vi "Calculate_Integrals.vi"(11 "SiPM Waveform":waveform(dbl)[](array[waveform])) -> (0 "Discrimination":string[](array[string]), 1 "Tail Integral":dbl[](array[numeric]), 2 "dt":dbl, 3 "Data Points":dbl[][](array[numeric]), 4 "Total Integral":dbl[](array[numeric]), 6 "Discrimination boolean":bool[](array[boolean]))   [LabVIEW 2015]
uses:
  ESA_Data_Analysis_Global_VIs.vi
  <vilib>/Analysis/NI_AALPro.lvlib
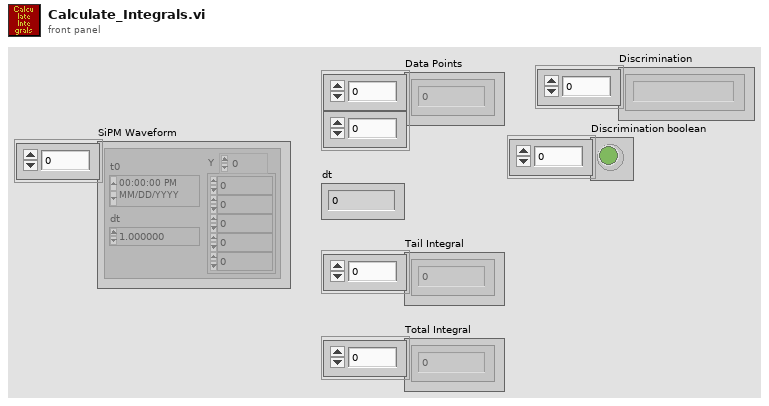
[diagram p1: front panel]
types:
  T1 = cluster{"Cursor.Cursor X1":dbl, "Cursor.Cursor Y1":dbl, "Cursor.Cursor X2":dbl, "Cursor.Cursor Y2":dbl}
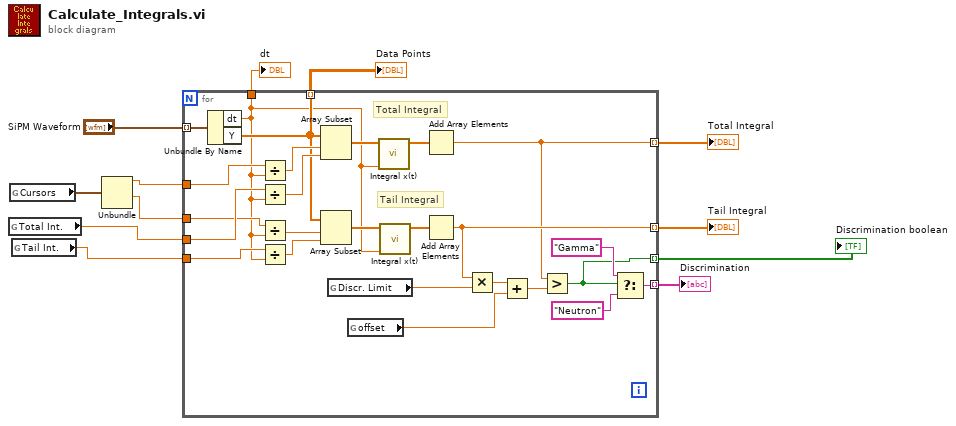
[diagram p0: block diagram]
diagram:
  n1 = global read "ESA_Data_Analysis_Global_VIs.vi" "Total Int."() -> (w4:dbl)
  n2 = global read "ESA_Data_Analysis_Global_VIs.vi" "Cursors"() -> (w7:T1)
  n3 = global read "ESA_Data_Analysis_Global_VIs.vi" "Tail Int."() -> (w3:dbl)
  n4 = Unbundle(w7) -> ("Cursor.Cursor X1"=w6:dbl, "Cursor.Cursor X2"=w5:dbl)  [unwired: 2 out]
  n5 = for {
    tunnel: "SiPM Waveform" -> [w33] mode=indexing
    tunnel: w6 -> [w32]
    tunnel: w4 -> [w31]
    tunnel: w5 -> [w30]
    tunnel: w3 -> [w29]
    tunnel: [w17] -> w12 mode=indexing
    tunnel: [w22] -> w11 mode=indexing
    tunnel: [w24] -> w9 mode=indexing
    tunnel: [w23] -> w10
    tunnel: [w14] -> w2 mode=indexing
    tunnel: [w13] -> w1 mode=indexing
    # "Total Integral"
    # "Tail Integral"
    n6 = Unbundle By Name(w33) -> ("dt"=w23:dbl, "Y"=w24:dbl[])
    n7 = Divide(x=w32, y=w23) -> (x/y=w37:dbl)
    n8 = Divide(x=w31, y=w23) -> (x/y=w36:dbl)
    n9 = Divide(x=w30, y=w23) -> (x/y=w34:dbl)
    n10 = Divide(x=w29, y=w23) -> (x/y=w35:dbl)
    n11 = Array Subset(array=w24, index=w37, length=w36) -> (w25:dbl[])
    n12 = Array Subset(array=w24, index=w34, length=w35) -> (w28:dbl[])
    n13 = global read "ESA_Data_Analysis_Global_VIs.vi" "Discr. Limit"() -> (w21:dbl)
    n14 = global read "ESA_Data_Analysis_Global_VIs.vi" "offset"() -> (w19:dbl)
    n15 = call <vilib>:"Integral x(t).vi"("dt"=w23, "X"=w25) -> ("Integral X"=w27:dbl[])  [unwired: 8 in, 1 out]
    n16 = call <vilib>:"Integral x(t).vi"("dt"=w23, "X"=w28) -> ("Integral X"=w26:dbl[])  [unwired: 8 in, 1 out]
    n17 = Add Array Elements(numeric array=w27) -> (sum=w17:dbl)
    n18 = Add Array Elements(numeric array=w26) -> (sum=w22:dbl)
    n19 = Multiply(x=w22, y=w21) -> (x*y=w20:dbl)
    n20 = Add(x=w20, y=w19) -> (x+y=w18:dbl)
    n21 = Greater?(x=w17, y=w18) -> (0:w13:bool)
    n22 = Select(t="Gamma", s=w13, f="Neutron") -> (s? t:f=w14:string)
  }
  "Total Integral" <- w12
  "Tail Integral" <- w11
  "dt" <- w10
  "Data Points" <- w9
  "Discrimination" <- w2
  "Discrimination boolean" <- w1
